vi "Data2Time.vi"(11 "data":T1={"year"="2015", "month"="1", "day"="1", "hour"="21", "minute"="23", "second"="5"}) -> (3 "Time":timestamp)   [LabVIEW 2017, in "UI_TimeSelector.xctl"]
uses:
  UI_TimeSelector/UI_TimeSelector.xctl
  UI_TimeSelector/Typedefs/INTERNAL-DATA.ctl
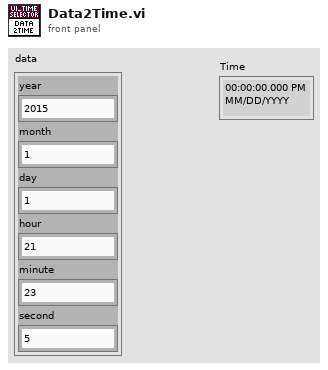
[diagram p1: front panel]
types:
  T1 = typedef "UI_TimeSelector.xctl/INTERNAL-DATA.ctl" = cluster{"year":string, "month":string, "day":string, "hour":string, "minute":string, "second":string}
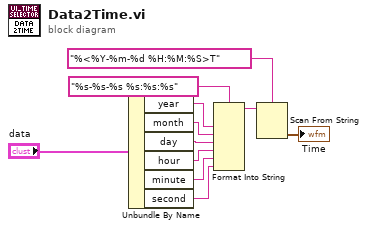
[diagram p0: block diagram]
diagram:
  n1 = Unbundle By Name("data") -> ("year"=w6:string, "month"=w5:string, "day"=w4:string, "hour"=w3:string, "minute"=w2:string, "second"=w1:string)
  n2 = Format Into String(format string="%s-%s-%s %s:%s:%s", w6, w5, w4, w3, w2, w1) -> (resulting string=w7:string)  [unwired: 2 in, 1 out]
  n3 = Scan From String(format string="%<%Y-%m-%d %H:%M:%S>T", input string=w7) -> (output 1=→"Time":timestamp)  [unwired: 3 in, 3 out]
